vi "UpDataResult.vi"(8 "error in (no error)":errorcluster, 9 "Time":dbl, 10 "UpDataResult":T1(array[cluster]), 11 "TestBench in":refnum<class "TestBench.lvclass">) -> (0 "error out":errorcluster, 3 "TestBench out":refnum<class "TestBench.lvclass">)   [LabVIEW 2019, in "TestBench.lvlib" / "TestBench.lvclass"]
uses:
  TestBench.lvclass
  TestBench.lvclass/TestBench.ctl
  TestEngine/TestEngine/Number of Steps.lvclass
  C:/Program Files (x86)/National Instruments/LabVIEW 2019/vi.lib/NI/Event Source Actor/Event Source/Event/Event.lvclass
  <vilib>/NI/Event Source Actor/Event Source/Event/Event.lvclass/Event.ctl
  UnitTestEngine/UnitTestEngine Messages/UpDataResult Msg/UpDataResult Msg.lvclass/UpDataResult Msg.ctl
  <vilib>/ActorFramework/Message Enqueuer/Message Enqueuer.lvclass/Message Enqueuer.ctl
  <vilib>/NI/Event Source Actor/Event Source/Event Source Messages/Generate Event Msg/Generate Event Msg.lvclass/Generate Event Msg.ctl
  <vilib>/ActorFramework/Message Enqueuer/Enqueue.vi
  UnitTestEngine/UnitTestEngine Messages/UpDataResult Msg/UpDataResult Msg.lvclass
  C:/Program Files (x86)/National Instruments/LabVIEW 2019/vi.lib/ActorFramework/Message/Message.lvclass
  <vilib>/NI/Event Source Actor/Event Source/Event Source Messages/Generate Event Msg/Generate Event Msg.lvclass
  <vilib>/ActorFramework/Message Priority Queue/Priority Enqueue.vi
  <vilib>/NI/Event Source Actor/Event Source/Event/Event.lvclass
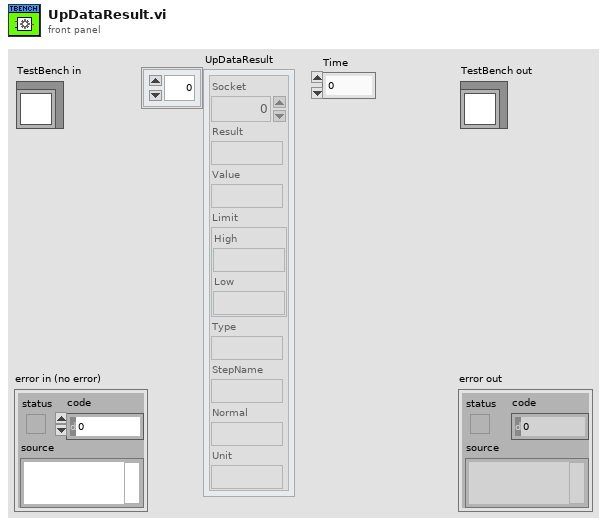
[diagram p1: front panel]
types:
  T1 = cluster{"Socket":i32, "Result":string, "Value":string, "Limit":cluster{"High":string, "Low":string}, "Type":string, "StepName":string, "Normal":string, "Unit":string}[]
  T2 = map{string, refnum<class "Message Enqueuer.lvclass">}
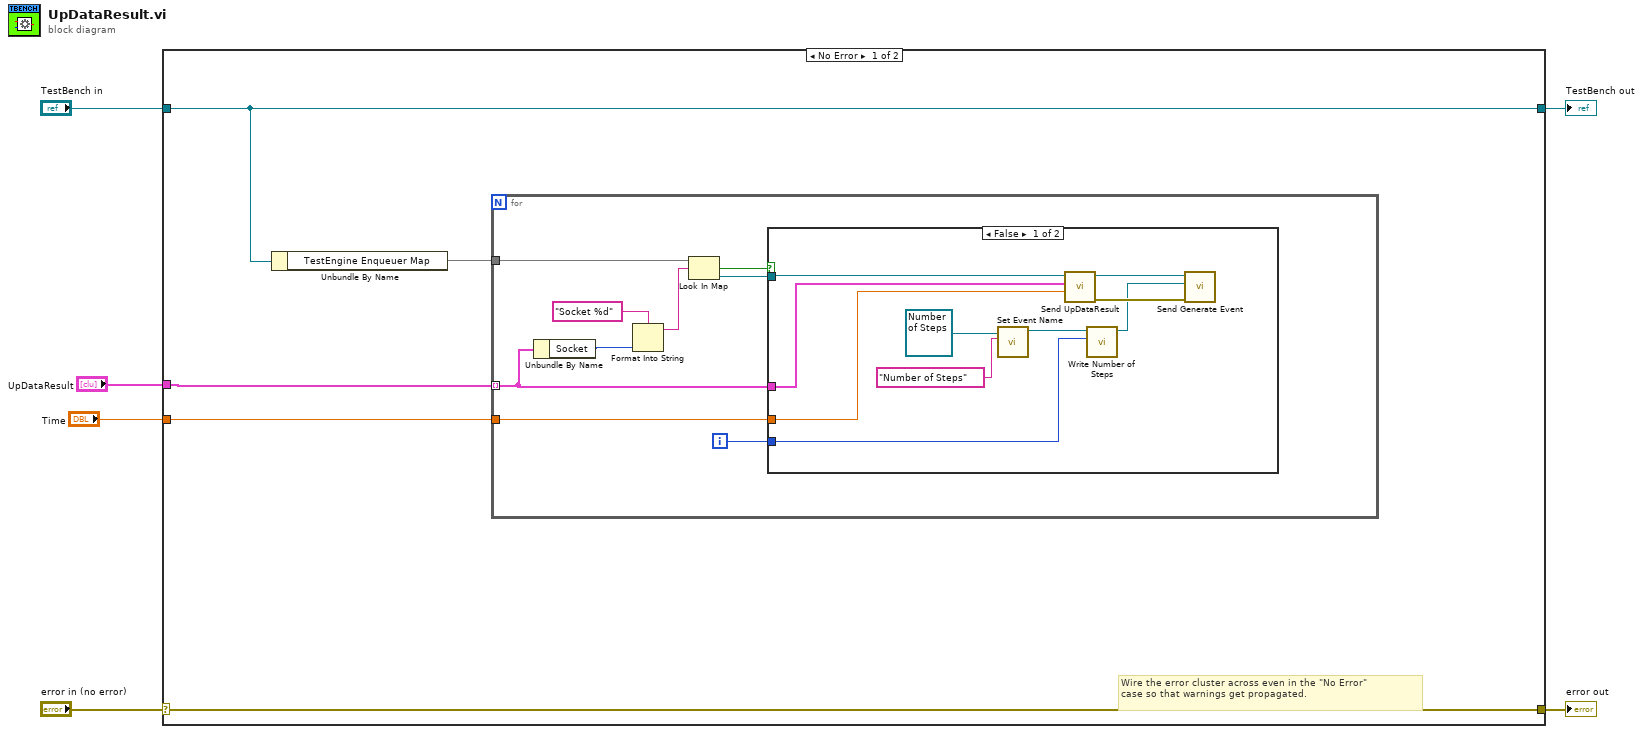
[diagram p0: block diagram]
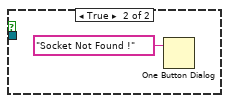
[diagram p2: hidden frame]
diagram:
  n1 = case shown="No Error" "error in (no error)" {
    selector: "error in (no error)" -> [w11 w33]
    tunnel: [w11 w33] -> w5
    tunnel: [w10 w32] -> w3
    tunnel: "TestBench in" -> [w10 w32]
    tunnel: "UpDataResult" -> [w8 _]
    tunnel: "Time" -> [w7 _]
    frame No Error {
      # "Wire the error cluster across even in the \"No Error\"\ncase so that warnings get propagated."
      n2 = Unbundle By Name(w10) -> ("TestEngine Enqueuer Map"=w9:T2)
      n3 = for {
        tunnel: w8 -> [w17] mode=indexing
        tunnel: w9 -> [w20]
        tunnel: w7 -> [w12]
        i -> [w13]
        n4 = Unbundle By Name(w17) -> ("Socket"=w15:i32)
        n5 = Format Into String(format string="Socket %d", w15) -> (resulting string=w14:string)  [unwired: 2 in, 1 out]
        n6 = Look In Map(map=w20, key=w14) -> (key not found?=w18:bool, value=w19:refnum<class "Message Enqueuer.lvclass">)  [unwired: 1 in]
        n7 = case shown="False" w18 {
          tunnel: w19 -> [w24 _]
          tunnel: w17 -> [w23 _]
          tunnel: w13 -> [w22 _]
          tunnel: w12 -> [w21 _]
          frame False {
            n8 = call <vilib>:"Set Event Name.vi"("Name (Generic)"="Number of Steps", "Event In"=refnum<class "Number of Steps.lvclass"> refnum ("TestEngine.lvlib:Number of Steps.lvclass")) -> ("Event Out"=w28:refnum<class "Number of Steps.lvclass">)  [unwired: 9 in]
            n9 = call "Send UpDataResult.vi"("Time"=w21, "UpDataResult"=w23, "Message Enqueuer"=w24) -> ("error out"=w30:errorcluster, "Message Enqueuer out"=w29:refnum<class "Message Enqueuer.lvclass">)  [unwired: 7 in]
            n10 = call-dynamic "Write Number of Steps.vi"("Number of Steps"=w22, "Number of Steps in"=w28) -> ("Number of Steps out"=w27:refnum<class "Number of Steps.lvclass">)  [unwired: 8 in, 1 out]
            n11 = call <vilib>:"Send Generate Event.vi"("Error In"=w30, "Event"=w27, "Event Source Address"=w29) -> ()  [unwired: 7 in, 2 out]
          }
          frame True {
            n12 = One Button Dialog(message="Socket Not Found !") -> ()  [unwired: 1 in, 1 out]
          }
        }
      }
    }
    frame Error {
    }
  }
  "error out" <- w5
  "TestBench out" <- w3
